vi "RunOperation.vi"(10 "Inputs":string[](array[string]), 11 "DiffVI in":refnum<class "DiffVI.lvclass">) -> (1 "Output/Failure":string, 2 "CLI Process Return Code":i32, 3 "DiffVI out":refnum<class "DiffVI.lvclass">)   [LabVIEW 2018, in "DiffVI.lvclass"]
uses:
  DiffVI.lvclass
  DiffVI.lvclass/DiffVI.ctl
  <vilib>/Utility/error.llb/DialogType.ctl
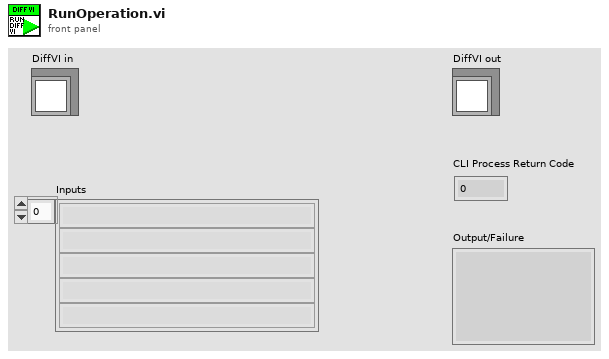
[diagram p1: front panel]
types:
  T1 = typedef "DialogType.ctl" = u16
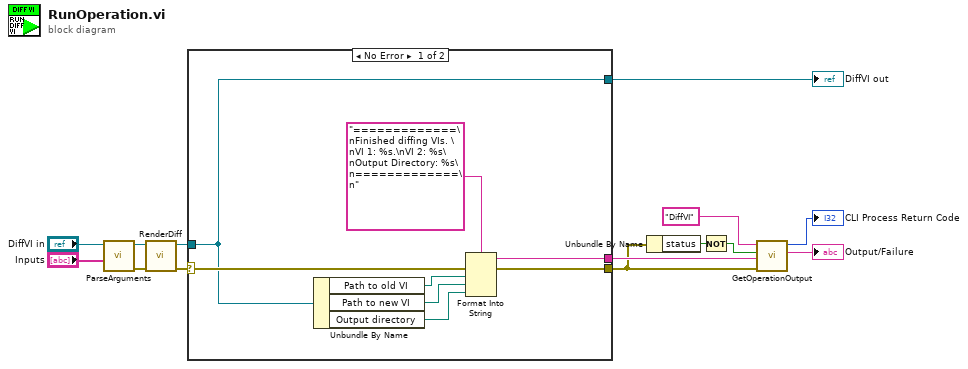
[diagram p0: block diagram]
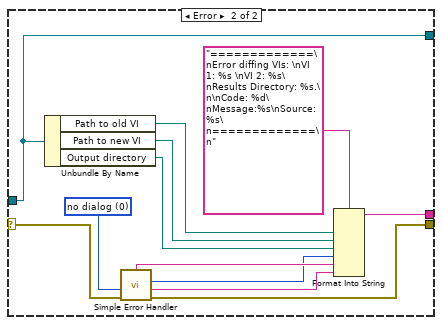
[diagram p2: hidden frame]
diagram:
  n1 = call "ParseArguments.vi"("Inputs"="Inputs", "DiffVI in"="DiffVI in") -> ("error out"=w13:errorcluster, "DiffVI out"=w10:refnum<class "DiffVI.lvclass">)  [unwired: 8 in]
  n2 = call "RenderDiff.vi"("error in (no error)"=w13, "DiffVI in"=w10) -> ("error out"=w14:errorcluster, "DiffVI out"=w9:refnum<class "DiffVI.lvclass">)  [unwired: 8 in]
  n3 = case shown="No Error" w14 {
    selector: w14 -> [w21 w33]
    tunnel: [w20 w34] -> w7
    tunnel: w9 -> [w19 w27]
    tunnel: [w19 w27] -> w8
    tunnel: [w15 w23] -> w6
    frame No Error {
      n4 = Unbundle By Name(w19) -> ("Path to old VI"=w18:path, "Path to new VI"=w17:path, "Output directory"=w16:path)
      n5 = Format Into String(format string="=============\nFinished diffing VIs. \nVI 1: %s.\nVI 2: %s\nOutput Directory: %s\n=============\n", error in=w21, w18, w17, w16) -> (resulting string=w20:string, error out=w15:errorcluster)  [unwired: 1 in]
    }
    frame Error {
      w32 = T1 0 items=["no dialog", "OK message", "continue or stop message", "OK message + warnings", "continue/stop + warnings"] ("type of dialog (OK msg:1)")
      n6 = Unbundle By Name(w27) -> ("Path to old VI"=w26:path, "Path to new VI"=w25:path, "Output directory"=w24:path)
      n7 = call <vilib>:"Simple Error Handler.vi"("type of dialog (OK msg:1)"=w32, "error in (no error)"=w33) -> ("code out"=w28:i32, "source out"=w29:string, "error out"=w23:errorcluster, "message"=w30:string)  [unwired: 3 in, 1 out]
      n8 = Format Into String(format string="=============\nError diffing VIs: \nVI 1: %s \nVI 2: %s\nResults Directory: %s.\n\nCode: %d\nMessage:%s\nSource: %s\n=============\n", w26, w25, w24, w28, w30, w29) -> (resulting string=w34:string)  [unwired: 2 in, 1 out]
    }
  }
  "DiffVI out" <- w8
  n9 = Unbundle By Name(w6) -> ("status"=w2:bool)
  n10 = Not(x=w2) -> (.not. x?=w1:bool)
  n11 = call <nishared>:"GetOperationOutput.vi"("error in (no error)"=w6, "Operation Output/Error In"=w7, "Operation succeeded?"=w1, "Operation Name"="DiffVI") -> ("Operation Output/Error Out"=→"Output/Failure":string, "CLI Process Return Code"=→"CLI Process Return Code":i32)  [unwired: 6 in]
